vi "oa_Check Params for Envelope Detection (Hz).vi"(6 "pulse/revolution (1)":i32=1, 7 "reset":bool, 8 "error in (no error)":errorcluster, 9 "span":dbl, 10 "center":dbl, 11 "dt":dbl) -> (0 "error out":errorcluster, 1 "span out":dbl, 2 "center out":dbl, 3 "dt out":dbl, 4 "pulse/revolution out":i32, 5 "reset out":bool)   [LabVIEW 2017, in "SoundVib_FaultAnalysis.lvlib"]
uses:
  <vilib>/addons/Sound and Vibration/Order Analysis/Fault Analysis/SoundVib_FaultAnalysis.lvlib
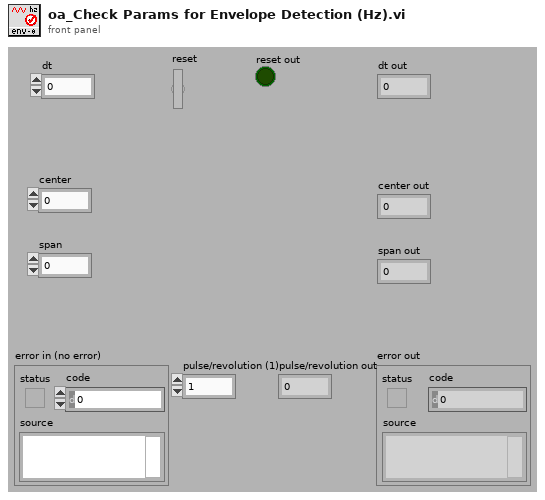
[diagram p1: front panel]
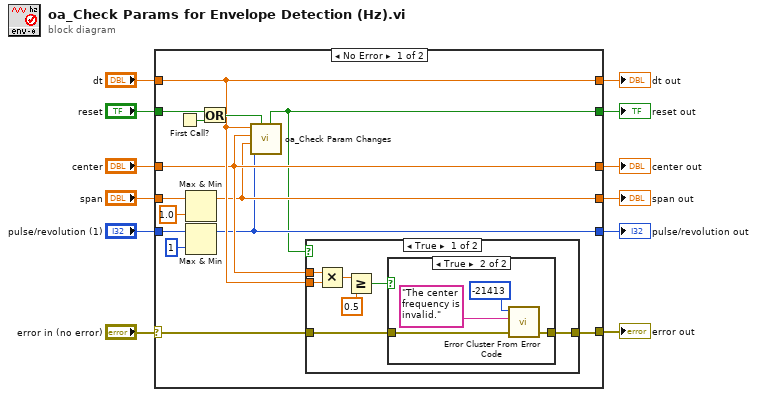
[diagram p0: block diagram]
diagram:
  n1 = case shown="No Error" "error in (no error)" {
    selector: "error in (no error)" -> [w26 w45]
    tunnel: [w25 w45] -> w11
    tunnel: "dt" -> [w21 w42]
    tunnel: "pulse/revolution (1)" -> [w18 w43]
    tunnel: "reset" -> [w23 w44]
    tunnel: [w13 w44] -> w8
    tunnel: [w15 w43] -> w7
    tunnel: [w21 w42] -> w6
    tunnel: "center" -> [w17 w41]
    tunnel: [w17 w41] -> w2
    tunnel: "span" -> [w19 w40]
    tunnel: [w16 w40] -> w3
    frame No Error {
      n2 = First Call?() -> (First Call?: T/F=w24:bool)
      n3 = Max & Min(x=w19, y=1.0) -> (max(x,y)=w16:dbl)  [unwired: 1 out]
      n4 = Max & Min(x=w18, y=1) -> (max(x,y)=w15:i32)  [unwired: 1 out]
      n5 = Or(x=w23, y=w24) -> (x .or. y?=w22:bool)
      n6 = call <vilib>:"oa_Check Param Changes.vi"("Reset?"=w22, "param4"=w15, "param3"=w16, "param2"=w17, "param1"=w21) -> ("Reset out"=w13:bool)  [unwired: 6 in]
      n7 = case shown="True" w13 {
        tunnel: w26 -> [w30 w39]
        tunnel: [w29 w39] -> w25
        tunnel: w21 -> [w28 _]
        tunnel: w17 -> [w27 _]
        frame True {
          n8 = Multiply(x=w27, y=w28) -> (x*y=w33:dbl)
          n9 = Greater Or Equal?(x=w33, y=0.5) -> (x >= y?=w31:bool)
          n10 = case shown="True" w31 {
            tunnel: w30 -> [w34 w38]
            tunnel: [w34 w35] -> w29
            frame False {
            }
            frame True {
              n11 = call <vilib>:"Error Cluster From Error Code.vi"("error in (no error)"=w38, "error message (\"\")"="The center frequency is invalid." ("error message (\"\")"), "error code (0)"=-21413) -> ("error out"=w35:errorcluster)  [unwired: 6 in]
            }
          }
        }
        frame False {
        }
      }
    }
    frame Error {
    }
  }
  "error out" <- w11
  "reset out" <- w8
  "pulse/revolution out" <- w7
  "dt out" <- w6
  "span out" <- w3
  "center out" <- w2
